vi "All sensors.vi"() -> ()   [LabVIEW 2022 SP3]
uses:
  <vilib>/DAQmx/write.llb/DAQmx Write (Digital Bool 1Line 1Point).vi
  <vilib>/DAQmx/create/channels.llb/DAQmx Create Channel (DO-Digital Output).vi
  <vilib>/DAQmx/miscellaneous.llb/DAQmx Fill In Error Info.vi
  <vilib>/DAQmx/create/channels.llb/DAQmx Create Channel (AI-Voltage-Basic).vi
  <vilib>/DAQmx/read.llb/DAQmx Read (Digital Bool 1Line 1Point).vi
  <vilib>/DAQmx/create/channels.llb/DAQmx Create Channel (DI-Digital Input).vi
  <vilib>/DAQmx/read.llb/DAQmx Read (Analog 1D DBL NChan 1Samp).vi
panel:
  in  "lines":tag
  out "LED panel ON":bool
  in  "VISA resource name 4":refnum<visa-resource-name>
  in  "VISA resource name 3":refnum<visa-resource-name>
  in  "VISA resource name 2":refnum<visa-resource-name>
  in  "VISA resource name":refnum<visa-resource-name>
  out "Food Distributor - ON":bool
  in  "lines - Food Distributor":tag
  in  "stop":bool
  out "x/y":dbl
  out "Thermometer":dbl(slide) scale=0.0..100.0
  out "x+y Temperature":dbl
  out "Turbidity Meter":dbl(knob) scale=0.0..8.0
  out "x-y Turbidity Level":dbl
  out "Temperature Sensor Reading 2":dbl
  out "LDR Reading":dbl
  in  "stop 4":bool
  in  "physical channels - Temperature, Turbidity Sensor":tag
  out "Water Pump - ON":bool
  in  "lines - Water Pump":tag
  in  "lines- Level Sensor":tag
  in  "stop 2":bool
  out "Water Level - LOW":bool
  # "e"
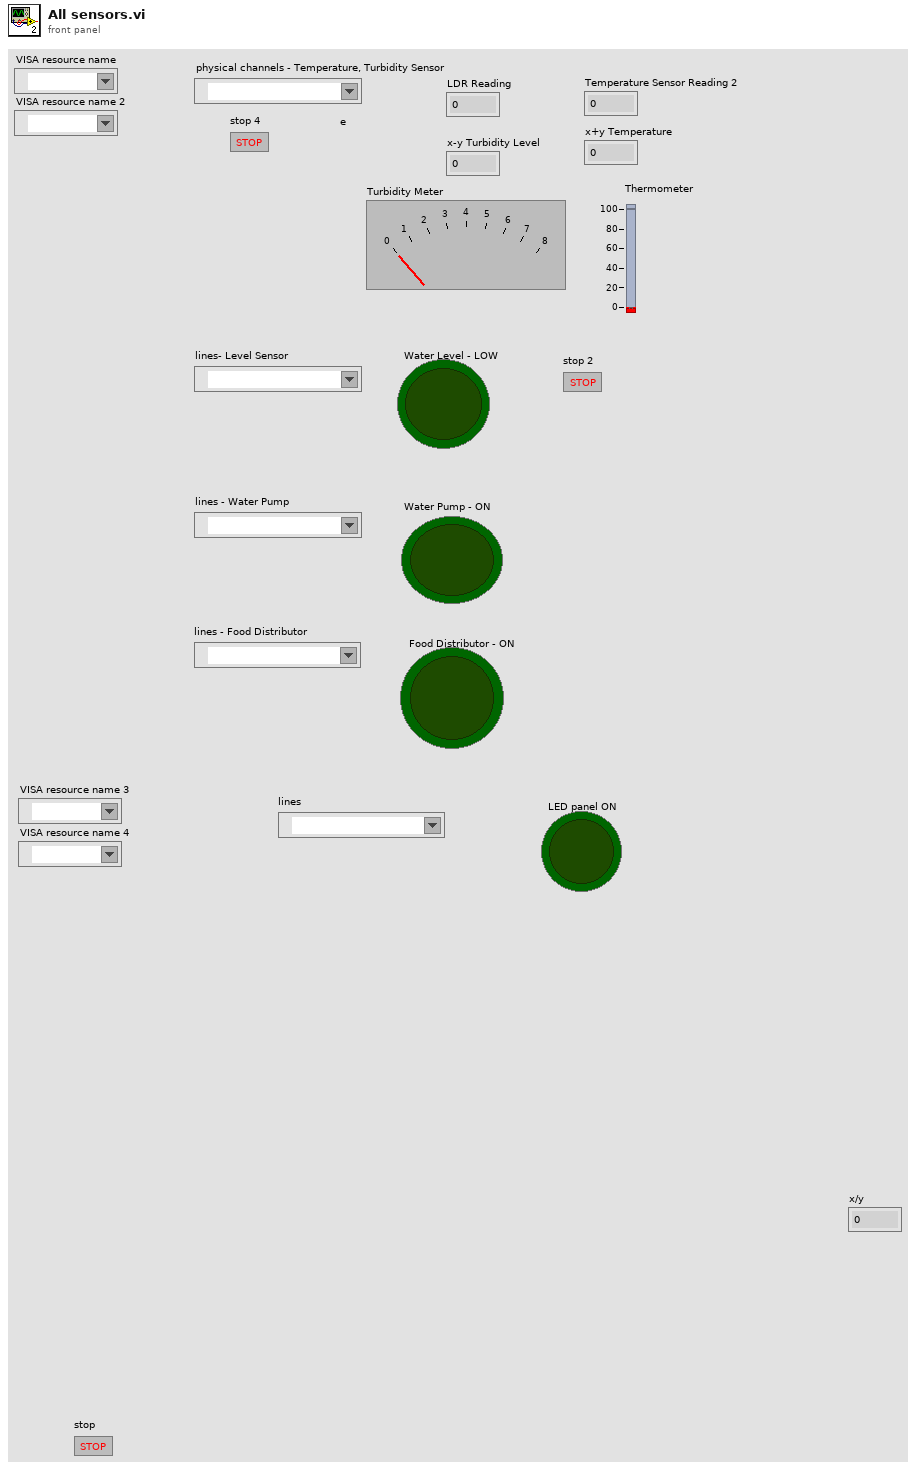
[diagram p1: front panel]
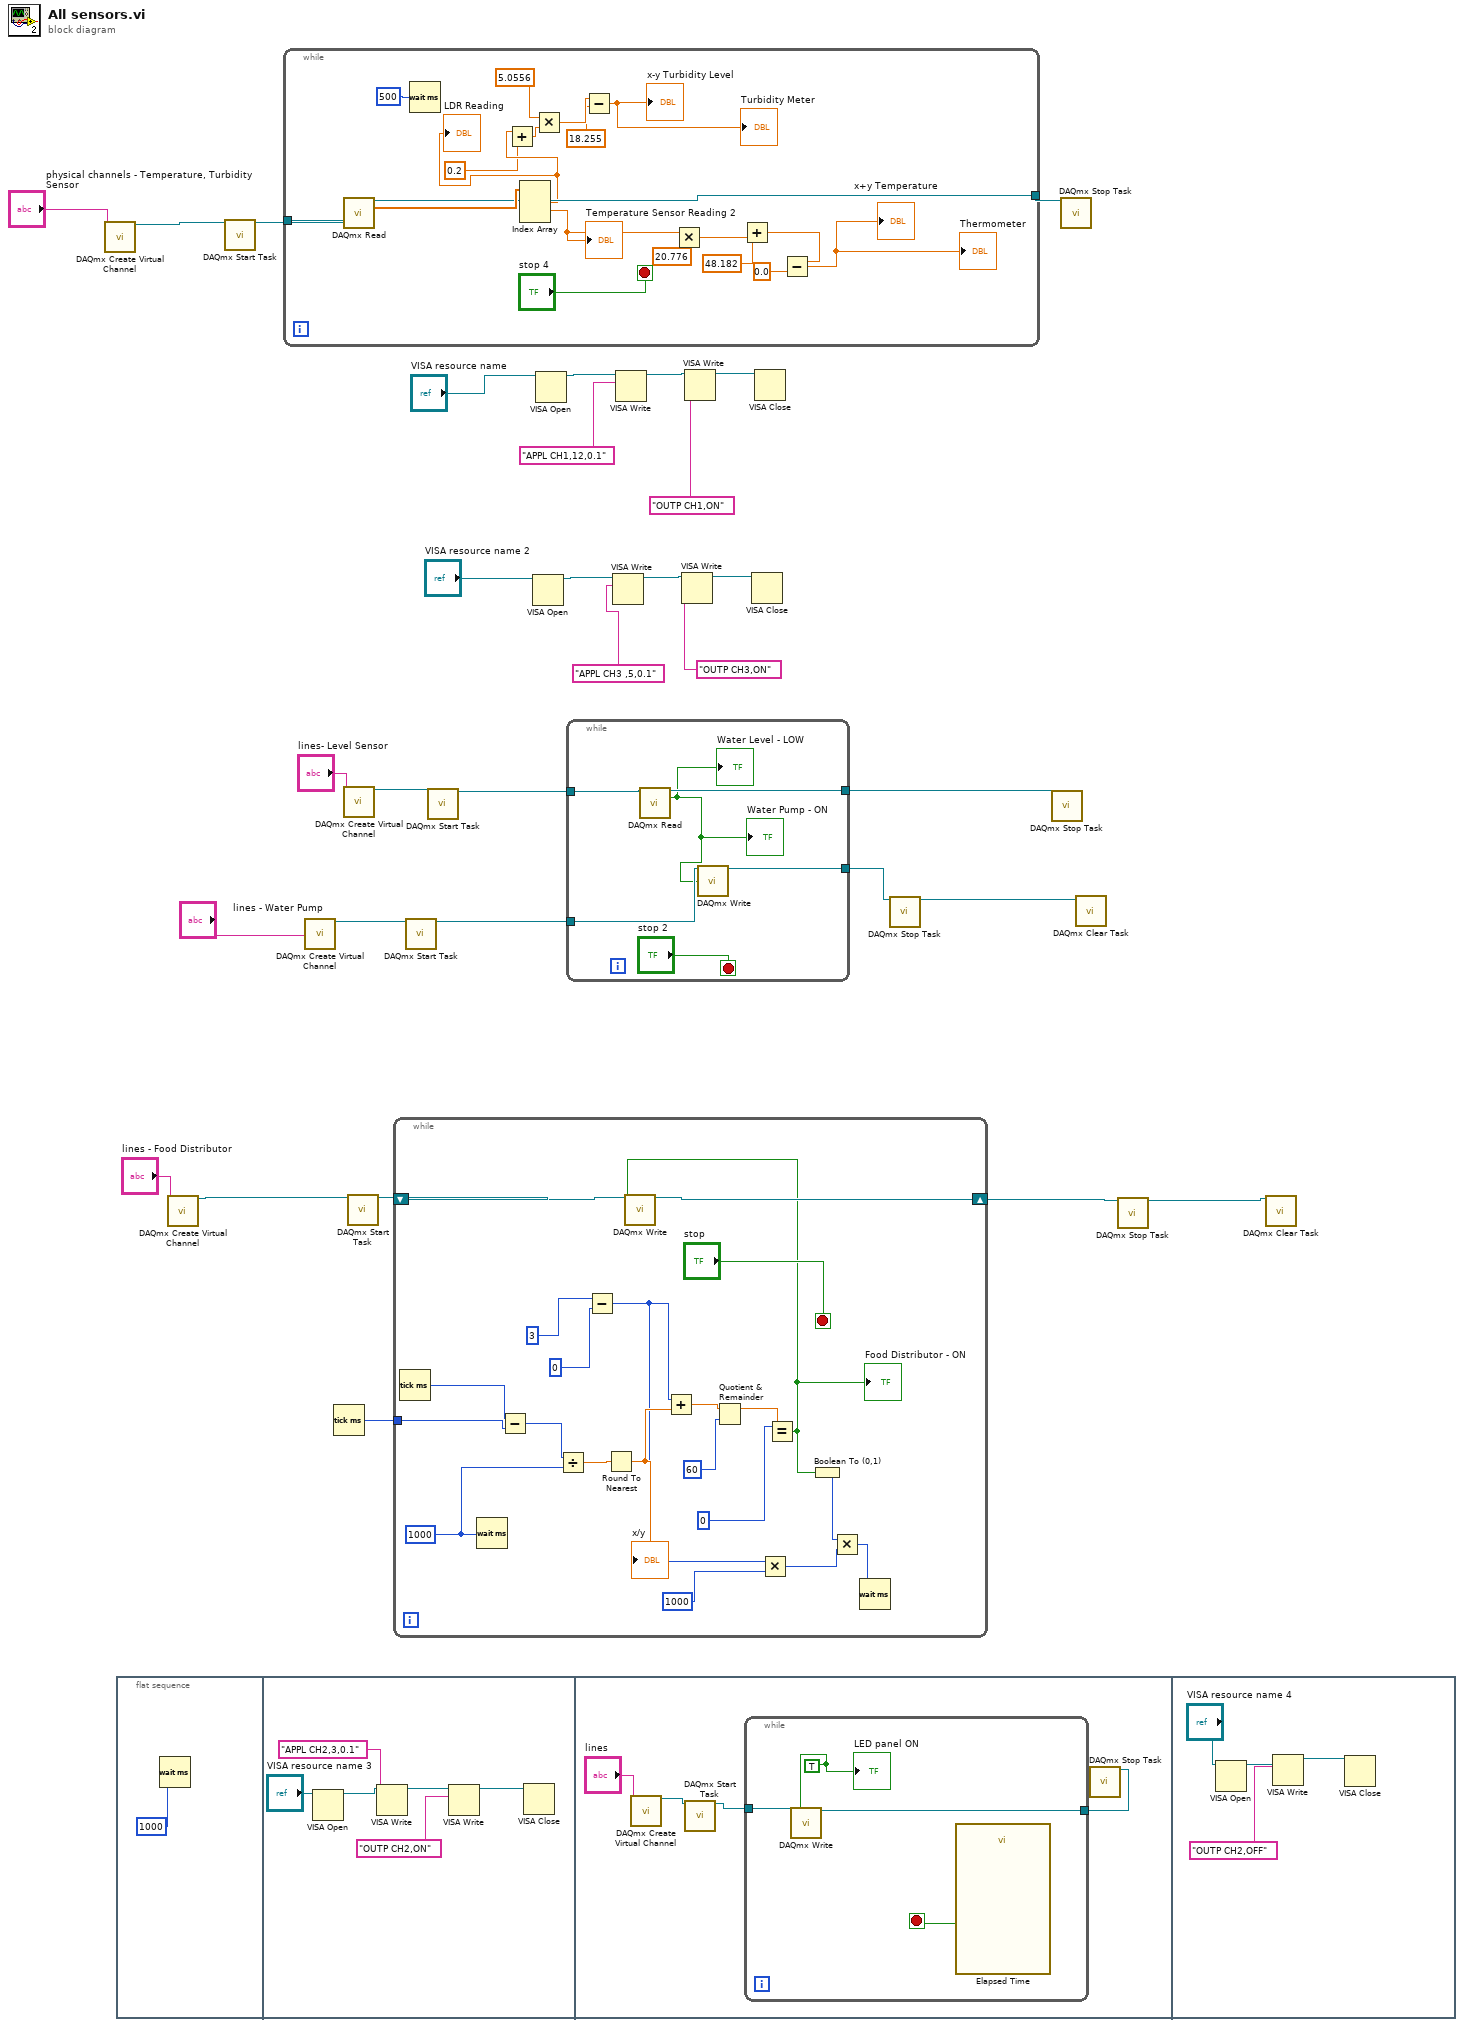
[diagram p0: block diagram]
diagram:
  n1 = call-poly <vilib>:"DAQmx Create Virtual Channel.vi"("physical channels"="physical channels - Temperature, Turbidity Sensor") -> ("task out"=w24:refnum<k21>)  [unwired: 13 in, 1 out]
  n2 = flat-sequence {
    frame #0 {
      n3 = Wait (ms)(milliseconds to wait=u32 1000 ("millisecond timer value")) -> ()  [unwired: 1 out]
    }
    frame #1 {
      n4 = VISA Open(VISA resource name="VISA resource name 3") -> (VISA resource name=w37:refnum<visa-resource-name>)  [unwired: 4 in, 1 out]
      n5 = VISA Write(VISA resource name=w37, write buffer="APPL CH2,3,0.1") -> (VISA resource name out=w36:refnum<visa-resource-name>)  [unwired: 1 in, 2 out]
      n6 = VISA Write(VISA resource name=w36, write buffer="OUTP CH2,ON") -> (VISA resource name out=w35:refnum<visa-resource-name>)  [unwired: 1 in, 2 out]
      n7 = VISA Close(VISA resource name=w35) -> ()  [unwired: 1 in, 1 out]
    }
    frame #2 {
      n8 = call-poly <vilib>:"DAQmx Create Virtual Channel.vi"("lines"="lines") -> ("task out"=w40:refnum<k21>)  [unwired: 13 in, 1 out]
      n9 = call <vilib>:"DAQmx Start Task.vi"("task/channels in"=w40) -> ("task out"=w42:refnum<k21>)  [unwired: 13 in, 1 out]
      n10 = while {
        tunnel: w42 -> [w46]
        tunnel: [w45] -> w41
        stop <- w44 stop-if-true
        w43 = TRUE
        n11 = call-poly <vilib>:"DAQmx Write.vi"("task/channels in"=w46, "data"=w43) -> ("task out"=w45:refnum<k21>)  [unwired: 11 in, 2 out]
        n12 = call "Elapsed Time"() -> ("Time has Elapsed"=w44:bool)  [unwired: 12 in, 7 out]
        "LED panel ON" <- w43
      }
      n13 = call <vilib>:"DAQmx Stop Task.vi"("task/channels in"=w41) -> ()  [unwired: 13 in, 2 out]
    }
    frame #3 {
      n14 = VISA Open(VISA resource name="VISA resource name 4") -> (VISA resource name=w49:refnum<visa-resource-name>)  [unwired: 4 in, 1 out]
      n15 = VISA Write(VISA resource name=w49, write buffer="OUTP CH2,OFF") -> (VISA resource name out=w48:refnum<visa-resource-name>)  [unwired: 1 in, 2 out]
      n16 = VISA Close(VISA resource name=w48) -> ()  [unwired: 1 in, 1 out]
    }
  }
  n17 = call-poly <vilib>:"DAQmx Create Virtual Channel.vi"("lines"="lines - Food Distributor") -> ("task out"=w16:refnum<k21>)  [unwired: 13 in, 1 out]
  n18 = call <vilib>:"DAQmx Start Task.vi"("task/channels in"=w24) -> ("task out"=w23:refnum<k21>)  [unwired: 13 in, 1 out]
  n19 = while {
    tunnel: w23 -> [w69]
    tunnel: [w66] -> w19
    stop <- "stop 4" stop-if-true
    n20 = call-poly <vilib>:"DAQmx Read.vi"("task/channels in"=w69) -> ("task out"=w66:refnum<k21>, "data"=w67:dbl[])  [unwired: 12 in, 1 out]
    n21 = Wait (ms)(milliseconds to wait=u32 500) -> ()  [unwired: 1 out]
    n22 = Index Array(array=w67) -> (element #1=w52:dbl, element #2=w61:dbl)  [unwired: 3 in, 1 out]
    "LDR Reading" <- w52
    "Temperature Sensor Reading 2" <- w61
    n23 = Add(x=w52, y=0.2) -> (x+y=w53:dbl)
    n24 = Multiply(x=5.0556, y=w53) -> (x*y=w64:dbl)
    n25 = Subtract(x=w64, y=18.255 ("x")) -> (x-y=→"x-y Turbidity Level" →"Turbidity Meter":dbl)
    n26 = Multiply(x=w61, y=20.776) -> (x*y=w59:dbl)
    n27 = Add(x=48.182, y=w59) -> (x+y=w56:dbl)
    n28 = Subtract(x=w56, y=0.0) -> (x-y=→"x+y Temperature" →"Thermometer":dbl)
  }
  n29 = call-poly <vilib>:"DAQmx Create Virtual Channel.vi"("lines"="lines - Water Pump") -> ("task out"=w27:refnum<k21>)  [unwired: 13 in, 1 out]
  n30 = Tick Count (ms)() -> (millisecond timer value=w14:u32)
  n31 = call-poly <vilib>:"DAQmx Create Virtual Channel.vi"("lines"="lines- Level Sensor") -> ("task out"=w31:refnum<k21>)  [unwired: 13 in, 1 out]
  n32 = call <vilib>:"DAQmx Start Task.vi"("task/channels in"=w16) -> ("task out"=w18:refnum<k21>)  [unwired: 13 in, 1 out]
  n33 = while {
    shift-right: [w89] -> w17
    shift-left: w18 -> [w90]
    tunnel: w14 -> [w86]
    stop <- "stop" stop-if-true
    w85 = 1000
    n34 = Tick Count (ms)() -> (millisecond timer value=w87:u32)
    n35 = Wait (ms)(milliseconds to wait=w85) -> ()  [unwired: 1 out]
    n36 = Subtract(x=w87, y=w86) -> (x-y=w84:u32)
    n37 = Divide(x=w84, y=w85) -> (x/y=w83:dbl)
    n38 = Subtract(x=3, y=0) -> (x-y=w71:i32)
    n39 = Round To Nearest(number=w83) -> (nearest integer value=w82:dbl)
    "x/y" <- w82
    n40 = Add(x=w71, y=w82) -> (x+y=w81:dbl)
    n41 = Quotient & Remainder(x=w81, y=60) -> (x-y*floor(x/y)=w79:dbl)  [unwired: 1 out]
    n42 = Multiply(x=w71, y=1000) -> (x*y=w73:i32)
    n43 = Equal?(x=0, y=w79) -> (x = y?=w70:bool)
    "Food Distributor - ON" <- w70
    n44 = call-poly <vilib>:"DAQmx Write.vi"("task/channels in"=w90, "data"=w70) -> ("task out"=w89:refnum<k21>)  [unwired: 11 in, 2 out]
    n45 = Boolean To (0,1)(Boolean=w70) -> (0, 1=w75:i16)
    n46 = Multiply(x=w75, y=w73) -> (x*y=w74:i32)
    n47 = Wait (ms)(milliseconds to wait=w74) -> ()  [unwired: 1 out]
  }
  n48 = call <vilib>:"DAQmx Start Task.vi"("task/channels in"=w27) -> ("task out"=w22:refnum<k21>)  [unwired: 13 in, 1 out]
  n49 = call <vilib>:"DAQmx Start Task.vi"("task/channels in"=w31) -> ("task out"=w29:refnum<k21>)  [unwired: 13 in, 1 out]
  n50 = VISA Open(VISA resource name="VISA resource name 2") -> (VISA resource name=w6:refnum<visa-resource-name>)  [unwired: 4 in, 1 out]
  n51 = VISA Open(VISA resource name="VISA resource name") -> (VISA resource name=w12:refnum<visa-resource-name>)  [unwired: 4 in, 1 out]
  n52 = while {
    tunnel: w29 -> [w95]
    tunnel: [w94] -> w28
    tunnel: w22 -> [w93]
    tunnel: [w92] -> w20
    stop <- "stop 2" stop-if-true
    n53 = call-poly <vilib>:"DAQmx Read.vi"("task/channels in"=w95) -> ("task out"=w94:refnum<k21>, "data"=w91:bool)  [unwired: 12 in, 1 out]
    "Water Level - LOW" <- w91
    "Water Pump - ON" <- w91
    n54 = call-poly <vilib>:"DAQmx Write.vi"("task/channels in"=w93, "data"=w91) -> ("task out"=w92:refnum<k21>)  [unwired: 11 in, 2 out]
  }
  n55 = VISA Write(VISA resource name=w6, write buffer="APPL CH3 ,5,0.1") -> (VISA resource name out=w4:refnum<visa-resource-name>)  [unwired: 1 in, 2 out]
  n56 = VISA Write(VISA resource name=w12, write buffer="APPL CH1,12,0.1") -> (VISA resource name out=w10:refnum<visa-resource-name>)  [unwired: 1 in, 2 out]
  n57 = VISA Write(VISA resource name=w4, write buffer="OUTP CH3,ON") -> (VISA resource name out=w3:refnum<visa-resource-name>)  [unwired: 1 in, 2 out]
  n58 = VISA Write(VISA resource name=w10, write buffer="OUTP CH1,ON") -> (VISA resource name out=w9:refnum<visa-resource-name>)  [unwired: 1 in, 2 out]
  n59 = VISA Close(VISA resource name=w3) -> ()  [unwired: 1 in, 1 out]
  n60 = VISA Close(VISA resource name=w9) -> ()  [unwired: 1 in, 1 out]
  n61 = call <vilib>:"DAQmx Stop Task.vi"("task/channels in"=w20) -> ("task out"=w21:refnum<k21>)  [unwired: 13 in, 1 out]
  n62 = call <vilib>:"DAQmx Stop Task.vi"("task/channels in"=w28) -> ()  [unwired: 13 in, 2 out]
  n63 = call <vilib>:"DAQmx Stop Task.vi"("task/channels in"=w19) -> ()  [unwired: 13 in, 2 out]
  n64 = call <vilib>:"DAQmx Clear Task.vi"("task in"=w21) -> ()  [unwired: 14 in, 1 out]
  n65 = call <vilib>:"DAQmx Stop Task.vi"("task/channels in"=w17) -> ("task out"=w15:refnum<k21>)  [unwired: 13 in, 1 out]
  n66 = call <vilib>:"DAQmx Clear Task.vi"("task in"=w15) -> ()  [unwired: 14 in, 1 out]
